vi "SetLoggerLevel.vi"(8 "error in (no error)":errorcluster, 10 "Level":T1=enum."WARNING", 11 "Logger in":refnum<class "Logger.lvclass">) -> (0 "error out":errorcluster, 3 "Logger out":refnum<class "Logger.lvclass">)   [LabVIEW 2022 SP3, in "Logger.lvlib" / "Logger.lvclass"]
uses:
  Logger.lvclass
  C:/Users/jakub/repos/gh/PythonWrapper/Source/PythonWrapper/PythonWrapper.lvclass
  _Level.ctl
  PythonWrapper/Source/PythonWrapper/PythonWrapper.lvclass/PythonWrapper.ctl
  Logger.lvclass/Logger.ctl
  PythonWrapper/Source/PythonWrapper/Read PythonSession.vi
  PythonWrapper/Source/PythonWrapper/Read ModulePath.vi
  Read Logger.vi
  Write Logger.vi
  Write Level.vi
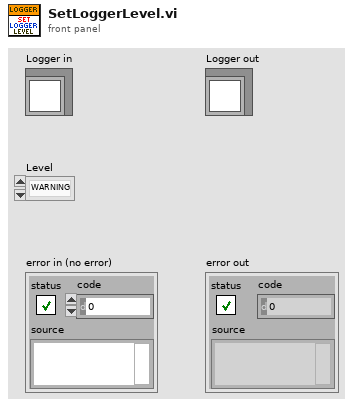
[diagram p1: front panel]
types:
  T1 = typedef "Logger.lvlib/Logger.lvclass/_Level.ctl" = enum16{"NOTSET", "DEBUG", "INFO", "WARNING", "ERROR", "CRITICAL"}
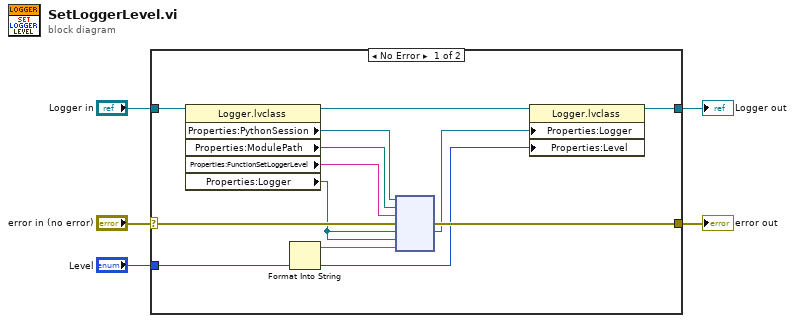
[diagram p0: block diagram]
diagram:
  n1 = case shown="No Error" "error in (no error)" {
    selector: "error in (no error)" -> [w15 w19]
    tunnel: [w14 w19] -> w4
    tunnel: [w10 w18] -> w2
    tunnel: "Logger in" -> [w17 w18]
    tunnel: "Level" -> [w8 _]
    frame No Error {
      n2 = property class="Logger.lvclass"(reference=w17) -> (reference out=w16:refnum<class "Logger.lvclass">, "Properties:PythonSession"=w13:refnum<k35>, "Properties:ModulePath"=w11:path, "Properties:FunctionSetLoggerLevel"=w12:string, "Properties:Logger"=w6:refnum<k38>)  [unwired: 1 in, 1 out]
      n3 = Format Into String(w8) -> (resulting string=w7:string)  [unwired: 3 in, 1 out]
      n4 = node(w13, w11, w12, w15, w6, w6, w7) -> (w14:errorcluster, w9:refnum<k38>)  [unwired: 2 in, 3 out]
      n5 = property class="Logger.lvclass"(reference=w16, "Properties:Logger"=w9, "Properties:Level"=w8) -> (reference out=w10:refnum<class "Logger.lvclass">)  [unwired: 1 in, 1 out]
    }
    frame Error {
    }
  }
  "error out" <- w4
  "Logger out" <- w2
